vi "line_initialise_collection.vi"(8 "error in (no error)":errorcluster, 11 "AnalysisRAPS in":refnum<class "AnalysisRAPS.lvclass">) -> (0 "error out":errorcluster, 3 "AnalysisRAPS out":refnum<class "AnalysisRAPS.lvclass">)   [LabVIEW 2010, in "AnalysisRAPS.lvclass"]
uses:
  AnalysisRAPS.lvclass
  AnalysisRAPS.lvclass/AnalysisRAPS.ctl
  common/classes/ImageCollection/ImageCollection/ImageCollection.lvclass
  common/classes/Image/Image/Image.lvclass
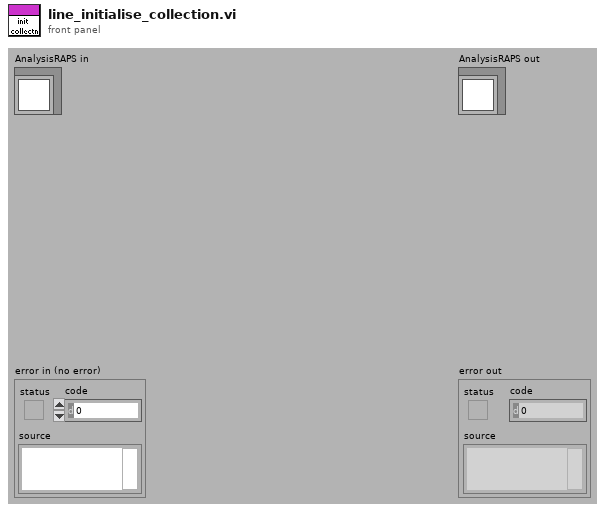
[diagram p1: front panel]
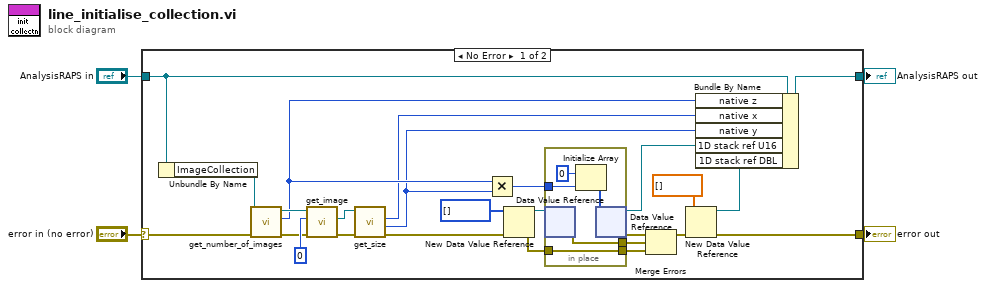
[diagram p0: block diagram]
diagram:
  n1 = case shown="No Error" "error in (no error)" {
    selector: "error in (no error)" -> [w11 w36]
    tunnel: [w7 w36] -> w3
    tunnel: [w17 w35] -> w1
    tunnel: "AnalysisRAPS in" -> [w18 w35]
    frame No Error {
      n2 = Unbundle By Name(w18) -> ("ImageCollection"=w29:refnum<class "ImageCollection.lvclass">)
      n3 = call-dynamic "get_number_of_images.vi"("error in (no error)"=w11, "ImageCollection in"=w29) -> ("error out"=w24:errorcluster, "size"=w16:i32, "ImageCollection out"=w28:refnum<class "ImageCollection.lvclass">)  [unwired: 7 in]
      n4 = call-dynamic "get_image.vi"("error in (no error)"=w24, "index"=0, "ImageCollection in"=w28) -> ("error out"=w25:errorcluster, "Image.lvclass"=w26:refnum<class "Image.lvclass">)  [unwired: 6 in, 1 out]
      n5 = call-dynamic "get_size.vi"("error in (no error)"=w25, "Image in"=w26) -> ("error out"=w22:errorcluster, "y resolution"=w10:i32, "x resolution"=w15:i32)  [unwired: 2 in, 5 out]
      n6 = Multiply(x=w16, y=w10) -> (x*y=w14:i32)
      n7 = New Data Value Reference(data value=u16[] [], error in=w22) -> (data value reference=w21:refnum<data-value>, error out=w13:errorcluster)
      n8 = in-place {
        in-place-border: [w34] -> w19
        in-place-border: w14 -> [w32]
        in-place-border: [w30] -> w12
        in-place-border: w13 -> [w30]
        n9 = in-place-dvr #1(w21) -> (w34:errorcluster)  [unwired: 1 out]
        n10 = Initialize Array(u16 0, w32) -> (w31:u16[])
        n11 = in-place-dvr #1(w31) -> (w6:refnum<data-value>, w20:errorcluster)
      }
      n12 = Merge Errors(w20, w19, w12) -> (w8:errorcluster)
      n13 = New Data Value Reference(data value=dbl[] [], error in=w8) -> (data value reference=w5:refnum<data-value>, error out=w7:errorcluster)
      n14 = Bundle By Name(cluster=w18, "native z"=w16, "native x"=w15, "native y"=w10, "1D stack ref U16"=w6, "1D stack ref DBL"=w5) -> (w17:refnum<class "AnalysisRAPS.lvclass">)
    }
    frame Error {
    }
  }
  "error out" <- w3
  "AnalysisRAPS out" <- w1
